vi "Stop Core.vi"(10 "final error code":i32, 11 "Signal_Gen in":refnum<class "Signal_Gen.lvclass">) -> (3 "Signal_Gen out":refnum<class "Signal_Gen.lvclass">)   [LabVIEW 2019, in "Signal_Gen.lvlib" / "Signal_Gen.lvclass"]
doc: "(<B>Filename</B>: Actor Framework.lvlib:Actor.lvclass:Stop Core.vi)\n\nDefines what the actor does before it stops. Use the <B>final error code</B> input to determine whether the actor shut down in response to an error.\n\nBy default, this method passes the Stop message along to all auto-stop nested actors. A descendant class may override this method to define additional behavior, such as shutting down any processes the actor initiated in its override of the Actor Core method."
uses:
  Signal_Gen.lvclass
  <vilib>/ActorFramework/Actor/Actor.lvclass
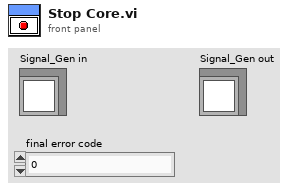
[diagram p1: front panel]
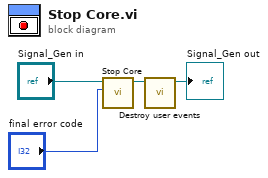
[diagram p0: block diagram]
diagram:
  n1 = call-parent "Stop Core.vi"("final error code"="final error code", "Actor in"="Signal_Gen in") -> ("Actor out"=w1:refnum<class "Signal_Gen.lvclass">)  [unwired: 9 in]
  n2 = call "Destroy user events.vi"("Signal_Gen in"=w1) -> ("Signal_Gen out"=→"Signal_Gen out":refnum<class "Signal_Gen.lvclass">)  [unwired: 9 in, 1 out]
